vi "generate_memtest_pulse.vi"(10 "external cmd sensitivity":dbl=20.0, 11 "memtest":T1={"Samples to Read"=2000, "Rate (Hz)"=20000.0, "Amplitude (mV/pA)"=10.0, "Offset (mV/pA)"=0.0, "Frequency (Hz)"=10.0, "duty cycle (%)"=50.0, "phase"=0.0} {"phase" format="%.2p"; "duty cycle (%)" format="%0.2f"}) -> (0 "view memtest":waveform(dbl)(graph), 3 "command memtest":waveform(dbl)(graph))   [LabVIEW 2019]
uses:
  controls/memtest_def.ctl
  <vilib>/measure/NI_MABase.lvlib
panel:
  out "size(s)":i32
  # "generate memtest pulse"
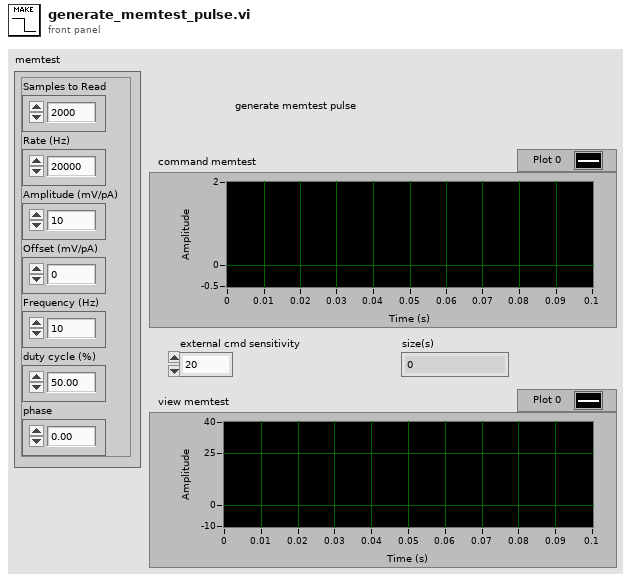
[diagram p1: front panel]
types:
  T1 = typedef "memtest_def.ctl" = cluster{"Samples to Read":i32, "Rate (Hz)":dbl, "Amplitude (mV/pA)":dbl, "Offset (mV/pA)":dbl, "Frequency (Hz)":dbl, "duty cycle (%)":dbl, "phase":dbl}
  T2 = enum16{"Sine Wave", "Triangle Wave", "Square Wave", "Sawtooth Wave"}
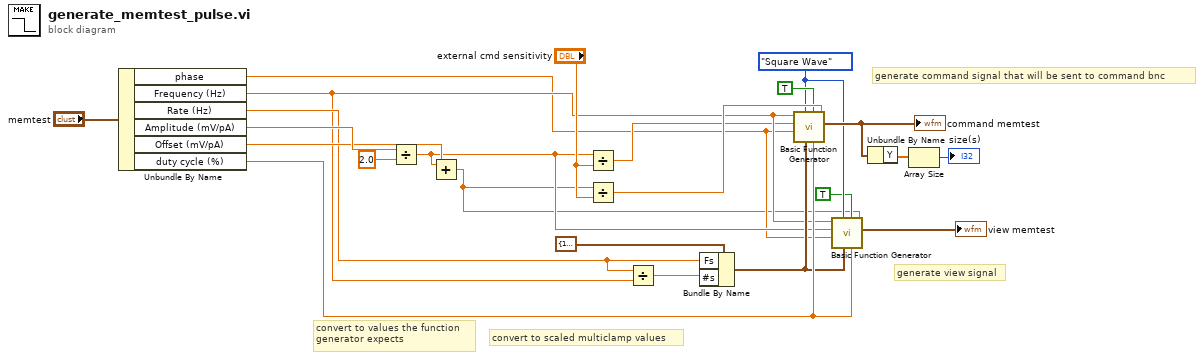
[diagram p0: block diagram]
diagram:
  w3 = T2."Square Wave" ("signal type")
  # "generate view signal"
  # "generate command signal that will be sent to command bnc"
  # "convert to values the function\ngenerator expects"
  # "convert to scaled multiclamp values"
  n1 = Unbundle By Name("memtest") -> ("phase"=w4:dbl, "Frequency (Hz)"=w7:dbl, "Rate (Hz)"=w15:dbl, "Amplitude (mV/pA)"=w22:dbl, "Offset (mV/pA)"=w20:dbl, "duty cycle (%)"=w9:dbl)
  n2 = Divide(x=w22, y=2.0) -> (x/y=w5:dbl)
  n3 = Add(x=w5, y=w20) -> (x+y=w1:dbl)
  n4 = Divide(x=w5, y="external cmd sensitivity") -> (x/y=w6:dbl)
  n5 = Divide(x=w1, y="external cmd sensitivity") -> (x/y=w19:dbl)
  n6 = Divide(x=w15, y=w7) -> (x/y=w16:dbl)
  n7 = Bundle By Name(cluster=cluster{"Fs":dbl, "#s":dbl} {"Fs"=1000.0, "#s"=1000.0} ("sampling info"), "Fs"=w15, "#s"=w16) -> (w8:cluster{"Fs":dbl, "#s":dbl})
  n8 = call <vilib>:"Basic Function Generator.vi"("offset"=w19, "square wave duty cycle (%)"=w9, "reset signal"=TRUE, "sampling info"=w8, "signal type"=w3, "phase"=w4, "amplitude"=w6, "frequency"=w7) -> ("signal out"=w14:waveform(dbl))  [unwired: 1 in, 2 out]
  "command memtest" <- w14
  n9 = call <vilib>:"Basic Function Generator.vi"("offset"=w1, "square wave duty cycle (%)"=w9, "reset signal"=TRUE, "sampling info"=w8, "signal type"=w3, "phase"=w4, "amplitude"=w5, "frequency"=w7) -> ("signal out"=→"view memtest":waveform(dbl))  [unwired: 1 in, 2 out]
  n10 = Unbundle By Name(w14) -> ("Y"=w11:dbl[])
  n11 = Array Size(array=w11) -> (size(s)=→"size(s)":i32)
